vi "raster navigation.vi"() -> ()   [LabVIEW 2010]
uses:
  <userlib>/Nanonis Prog Interface V5/Nanonis Prog Interface.lvlib
panel:
  out "Backwards Capacitance":dbl[][](graph)
  out "Backwards Delta":dbl[][](graph)
  out "Forwards Delta":dbl[][](graph)
  in  "Pixels per Backwards Row":u16=500
  in  "Pixels per Forward Row":u16=500
  in  "Vertical Direction":enum16{"X +", "X -", "Y +", "Y -"}(ring)
  out "Forwards Capacitance":dbl[][](graph)
  in  "Horizontal Direction":enum16{"X +", "X -", "Y +", "Y -"}(ring)
  out "Delta":cluster{"index":i32, sgl}[](graph)
  in  "Number of Steps":u16=500
  out "Capacitance":cluster{"index":i32, sgl}[](graph)
  in  "Frequency (Hz)":sgl=250.0
  in  "Amplitude (V)":sgl=150.0
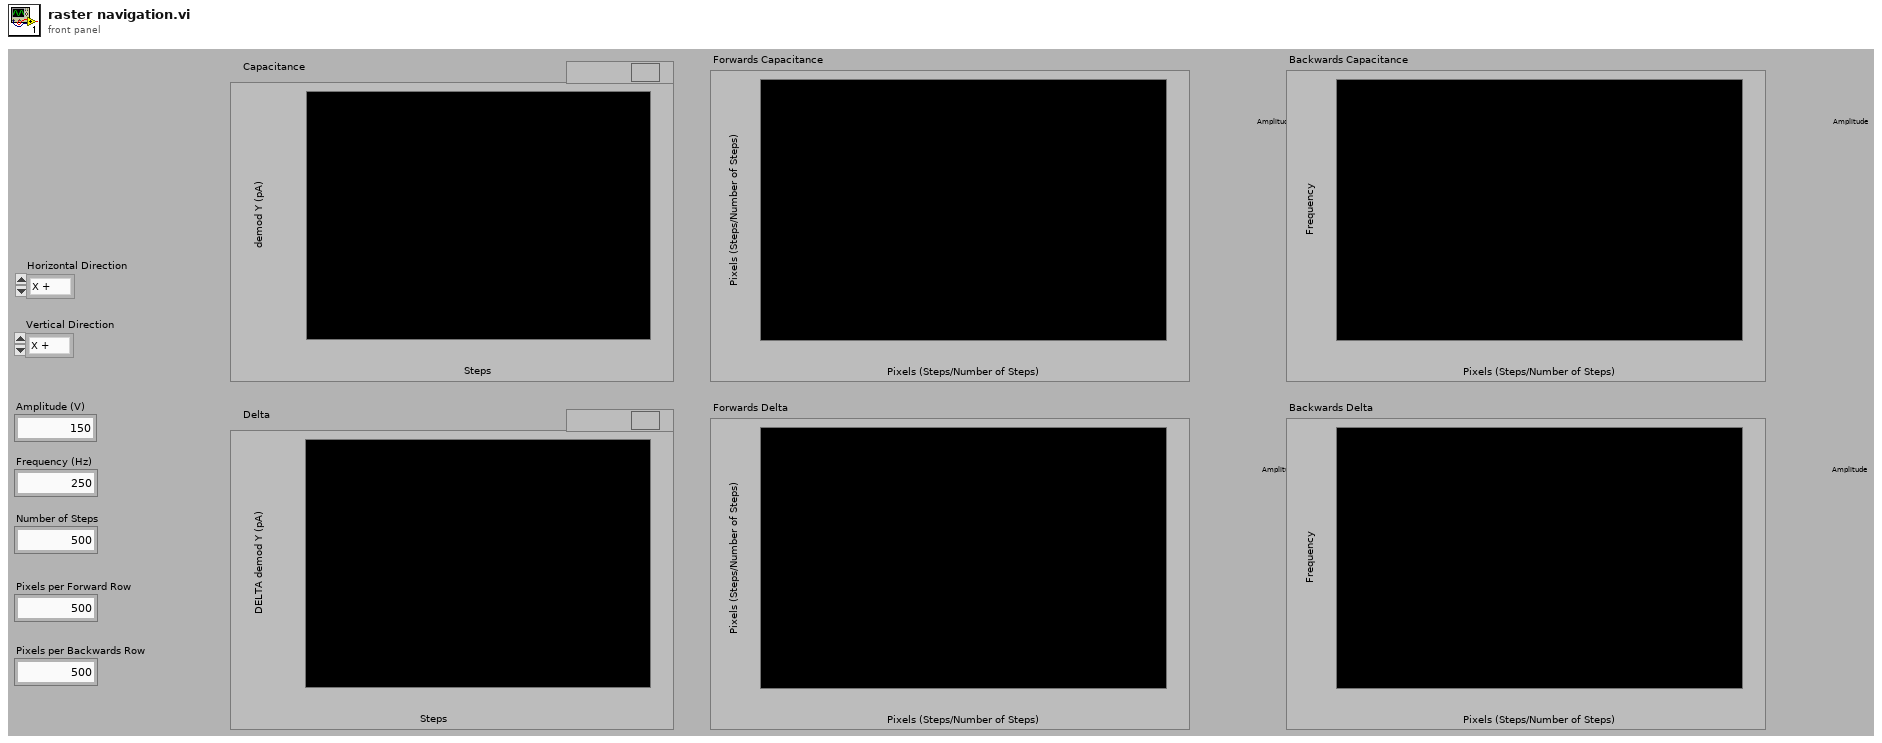
[diagram p1: front panel]
types:
  T1 = enum8{"Group 1", "Group 2", "Group 3", "Group 4", "Group 5", "Group 6"}
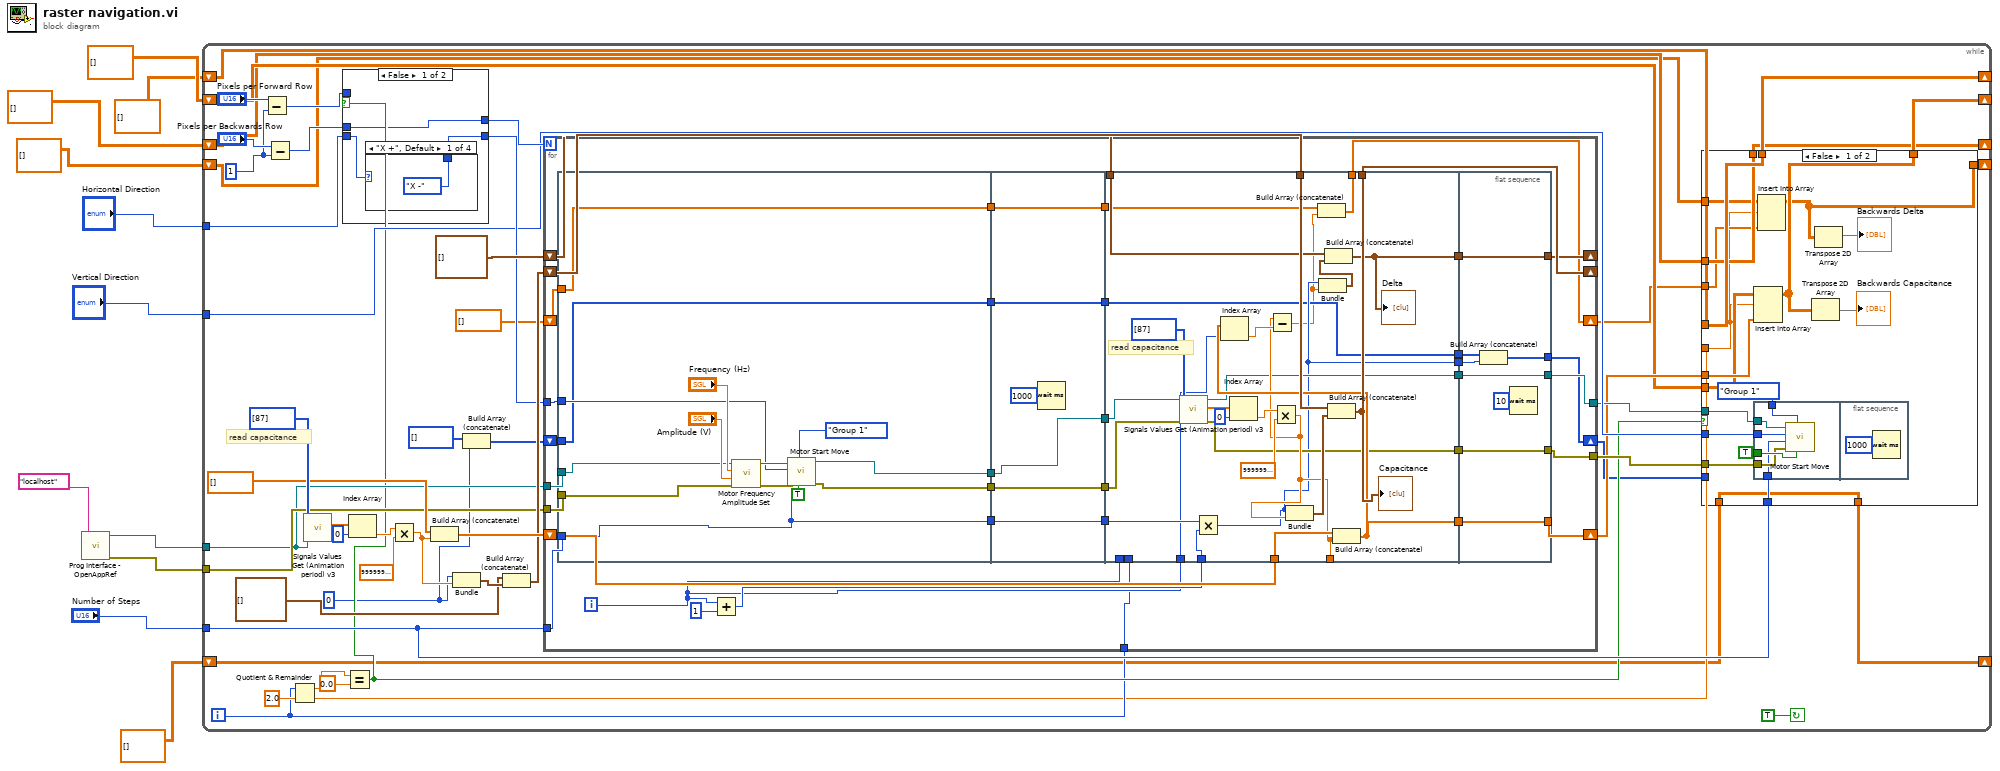
[diagram p0: block diagram]
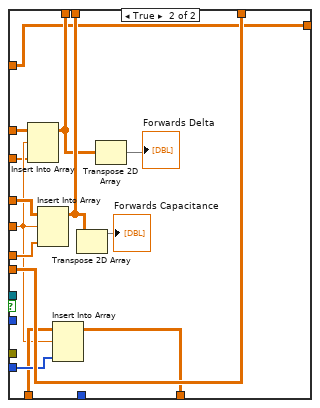
[diagram p2: hidden frame]
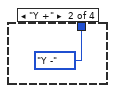
[diagram p3: hidden frame]
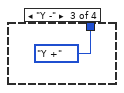
[diagram p4: hidden frame]
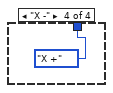
[diagram p5: hidden frame]
diagram:
  n1 = call <userlib>:"Prog Interface - OpenAppRef.vi"("Machine name (local machine IP)"="localhost" ("machine name (localhost)")) -> ("Error out"=w10:errorcluster, "Application reference"=w9:refnum<vi>)  [unwired: 5 in]
  n2 = while {
    tunnel: w10 -> [w50]
    tunnel: w9 -> [w49]
    tunnel: "Horizontal Direction" -> [w42]
    tunnel: "Number of Steps" -> [w32]
    tunnel: "Vertical Direction" -> [w35]
    shift-right: [w29] -> _
    shift-left: dbl[][] [] ("2D array") -> [w25]
    shift-right: [w24] -> _
    shift-left: dbl[][] [] ("2D array") -> [w27]
    shift-right: [w19] -> _
    shift-left: dbl[][] [] ("2D array") -> [w18]
    shift-right: [w14] -> _
    shift-left: dbl[][] [] ("2D array") -> [w15]
    shift-right: [w12] -> _
    shift-left: dbl[][] [] ("2D array") -> [w13]
    i -> [w28]
    stop <- TRUE continue-if-true
    w36 = u16 1 ("y")
    w23 = 0 ("index")
    # "read capacitance"
    n3 = Subtract(x="Pixels per Forward Row", y=w36) -> (x-y=w39:u16)
    n4 = Subtract(x="Pixels per Backwards Row", y=w36) -> (x-y=w37:u16)
    n5 = Quotient & Remainder(x=w28, y=2.0) -> (x-y*floor(x/y)=w43:dbl, floor(x/y)=w26:dbl)
    n6 = call <userlib>:"Signals Values Get (Animation period) v3.vi"("Signals indexes (0-127)"=i8[] [87], "Application ref in"=w49) -> ("Signals Values"=w59:sgl[])  [unwired: 6 in, 2 out]
    n7 = Equal?(x=w43, y=0.0) -> (x = y?=w31:bool)
    n8 = case shown="False" w31 {
      tunnel: [w103 w108] -> w46
      tunnel: w37 -> [w103 _]
      tunnel: w42 -> [w102 w109]
      tunnel: [w101 w109] -> w41
      tunnel: w39 -> [_ w108]
      frame False {
        n9 = case shown="\"X +\", Default" w102 {
          tunnel: [enum16{"X +", "X -", "Y +", "Y -"}."X -" ("Horizontal Direction 2") enum16{"X +", "X -", "Y +", "Y -"}."Y -" ("Horizontal Direction 2") enum16{"X +", "X -", "Y +", "Y -"}."Y +" ("Horizontal Direction 2") enum16{"X +", "X -", "Y +", "Y -"}."X +" ("Horizontal Direction 2")] -> w101
          frame "X +", Default {
          }
          frame "Y +" {
          }
          frame "Y -" {
          }
          frame "X -" {
          }
        }
      }
      frame True {
      }
    }
    n10 = Index Array(array=w59, index=0) -> (element=w58:sgl)
    n11 = Multiply(x=w58, y=sgl 1000000000000.0) -> (x*y=w54:sgl)
    n12 = Build Array (concatenate)(sgl[] [], w54) -> (w55:sgl[])
    n13 = Bundle("index"=w23, w54) -> (w53:cluster{"index":i32, sgl})  [unwired: 1 in]
    n14 = Build Array (concatenate)(i32[] [] ("array"), w23) -> (w21:i32[])
    n15 = Build Array (concatenate)(cluster{i32, sgl}[] [], w53) -> (w52:cluster{"index":i32, sgl}[])
    n16 = for {
      N: w46 -> [_]
      shift-right: [w143] -> _
      shift-left: w52 -> [w142]
      shift-right: [w141] -> w30
      shift-left: w55 -> [w140]
      tunnel: w49 -> [w136]
      tunnel: w50 -> [w135]
      shift-right: [w129] -> _
      shift-left: cluster{i32, sgl}[] [] -> [w128]
      tunnel: w41 -> [w127]
      tunnel: w32 -> [w124]
      tunnel: [w123] -> w34
      tunnel: [w122] -> w33
      tunnel: w28 -> [w120]
      shift-right: [w114] -> w20
      shift-left: w21 -> [w119]
      shift-right: [w110] -> w16
      shift-left: sgl[] [] ("array") -> [w113]
      i -> [w121]
      n17 = flat-sequence {
        tunnel: [w148] -> w145
        tunnel: w136 -> [w151]
        tunnel: w135 -> [w154]
        tunnel: [w153] -> w134
        tunnel: [w152] -> w133
        tunnel: w127 -> [w150]
        tunnel: w124 -> [w148]
        tunnel: w119 -> [w147]
        tunnel: [w147] -> w115
        tunnel: w113 -> [w146]
        tunnel: [w146] -> w111
        tunnel: w145 -> [w164]
        tunnel: [w164] -> w144
        tunnel: w134 -> [w163]
        tunnel: w133 -> [w162]
        tunnel: [w162] -> w132
        tunnel: [w163] -> w131
        tunnel: [w161] -> w116
        tunnel: w115 -> [w161]
        tunnel: [w160] -> w112
        tunnel: w111 -> [w160]
        tunnel: [w185] -> w143
        tunnel: w137 -> [w187]
        tunnel: w144 -> [w182]
        tunnel: w142 -> [w184]
        tunnel: w140 -> [w183]
        tunnel: [w176] -> _
        tunnel: [w179] -> w139
        tunnel: w132 -> [w181]
        tunnel: w131 -> [w180]
        tunnel: w121 -> [w178]
        tunnel: [w173] -> w130
        tunnel: w128 -> [w174]
        tunnel: [w172] -> w126
        tunnel: [w171] -> w125
        tunnel: w121 -> [_]
        tunnel: w120 -> [_]
        tunnel: [w170] -> w118
        tunnel: [w169] -> w117
        tunnel: w116 -> [w169]
        tunnel: w112 -> [w167]
        tunnel: [w166] -> w110
        tunnel: [w200] -> w141
        tunnel: w139 -> [w200]
        tunnel: w130 -> [w198]
        tunnel: [w198] -> w129
        tunnel: w126 -> [w197]
        tunnel: [w197] -> w123
        tunnel: w125 -> [w196]
        tunnel: [w196] -> w122
        tunnel: w118 -> [w195]
        tunnel: w117 -> [w194]
        tunnel: [w193] -> w114
        frame #0 {
          n18 = call <userlib>:"Motor Frequency Amplitude Set.vi"("Error in (no error)"=w154, "Amplitude (V) (NaN=no change)"="Amplitude (V)", "Frequency (Hz) (NaN=no change)"="Frequency (Hz)", "Application ref in"=w151) -> ("Error out"=w155:errorcluster, "Application ref out"=w156:refnum<vi>)  [unwired: 6 in]
          n19 = call <userlib>:"Motor Start Move.vi"("Wait until finished? (F)"=TRUE, "Group"=T1."Group 1", "Error in (no error)"=w155, "Number of steps"=w148, "Direction"=w150, "Application ref in"=w156) -> ("Error out"=w152:errorcluster, "Application ref out"=w153:refnum<vi>)  [unwired: 3 in]
        }
        frame #1 {
          n20 = Wait (ms)(milliseconds to wait=u32 1000) -> ()  [unwired: 1 out]
        }
        frame #2 {
          # "read capacitance"
          n21 = call <userlib>:"Signals Values Get (Animation period) v3.vi"("error in (no error)"=w181, "Signals indexes (0-127)"=i8[] [87], "Application ref in"=w180) -> ("error out"=w171:errorcluster, "Signals Values"=w190:sgl[], "Application ref out"=w172:refnum<vi>)  [unwired: 5 in]
          n22 = Multiply(x=w182, y=w187) -> (x*y=w170:i32)
          n23 = Index Array(array=w190, index=0) -> (element=w189:sgl)
          n24 = Multiply(x=w189, y=sgl 1000000000000.0) -> (x*y=w176:sgl)
          n25 = Bundle(w170, w176) -> (w186:cluster{i32, sgl})  [unwired: 1 in]
          n26 = Build Array (concatenate)(w184, w186) -> (w185:cluster{"index":i32, sgl}[])
          "Capacitance" <- w185
          n27 = Build Array (concatenate)(w183, w176) -> (w179:sgl[])
          n28 = Index Array(array=w179, index=w178) -> (element=w177:sgl)
          n29 = Subtract(x=w176, y=w177) -> (x-y=w168:sgl)
          n30 = Build Array (concatenate)(w167, w168) -> (w166:sgl[])
          n31 = Bundle(w170, w168) -> (w175:cluster{i32, sgl})  [unwired: 1 in]
          n32 = Build Array (concatenate)(w174, w175) -> (w173:cluster{i32, sgl}[])
          "Delta" <- w173
        }
        frame #3 {
          n33 = Build Array (concatenate)(w194, w195) -> (w193:i32[])
          n34 = Wait (ms)(milliseconds to wait=u32 10) -> ()  [unwired: 1 out]
        }
      }
      n35 = Add(x=w121, y=u16 1) -> (x+y=w137:i32)
    }
    n36 = case shown="False" w31 {
      tunnel: w35 -> [w77 _]
      tunnel: w34 -> [w76 _]
      tunnel: w33 -> [w75 _]
      tunnel: w32 -> [w74 _]
      tunnel: w30 -> [w72 w100]
      tunnel: w25 -> [w73 w99]
      tunnel: [w73 w92] -> w29
      tunnel: w26 -> [w64 w91]
      tunnel: w27 -> [w71 w98]
      tunnel: [w67 w98] -> w24
      tunnel: w20 -> [_ w97]
      tunnel: [w70 w96] -> w19
      tunnel: w18 -> [w70 w95]
      tunnel: w16 -> [w65 w90]
      tunnel: w15 -> [w66 w89]
      tunnel: [w66 w88] -> w14
      tunnel: w13 -> [w63 w87]
      tunnel: [w62 w87] -> w12
      frame False {
        n37 = Insert Into Array(array=w71, index (row)=w64, new element=w72) -> (w67:dbl[][])  [unwired: 1 in]
        n38 = flat-sequence {
          tunnel: T1."Group 1" ("Group") -> [w85]
          tunnel: TRUE ("Wait until finished? (F)") -> [w84]
          tunnel: w77 -> [w83]
          tunnel: w76 -> [w82]
          tunnel: w75 -> [w81]
          tunnel: w74 -> [w80]
          frame #0 {
            n39 = call <userlib>:"Motor Start Move.vi"("Wait until finished? (F)"=w84, "Group"=w85, "Error in (no error)"=w81, "Number of steps"=w80, "Direction"=w83, "Application ref in"=w82) -> ()  [unwired: 3 in, 2 out]
          }
          frame #1 {
            n40 = Wait (ms)(milliseconds to wait=u32 1000) -> ()  [unwired: 1 out]
          }
        }
        n41 = Insert Into Array(array=w63, index (row)=w64, new element=w65) -> (w62:dbl[][])  [unwired: 1 in]
        n42 = Transpose 2D Array(2D array=w67) -> (transposed array=→"Backwards Capacitance":dbl[][])
        n43 = Transpose 2D Array(2D array=w62) -> (transposed array=→"Backwards Delta":dbl[][])
      }
      frame True {
        n44 = Insert Into Array(array=w89, index (row)=w91, new element=w90) -> (w88:dbl[][])  [unwired: 1 in]
        n45 = Insert Into Array(array=w99, index (row)=w91, new element=w100) -> (w92:dbl[][])  [unwired: 1 in]
        n46 = Insert Into Array(array=w95, index (row)=w91, new element=w97) -> (w96:dbl[][])  [unwired: 1 in]
        n47 = Transpose 2D Array(2D array=w92) -> (transposed array=→"Forwards Capacitance":dbl[][])
        n48 = Transpose 2D Array(2D array=w88) -> (transposed array=→"Forwards Delta":dbl[][])
      }
    }
  }
